vi "Autotest_Instr.vi"(8 "error in (no error)":errorcluster caption="entrée d'erreur (pas d'erreur)", 11 "Class Instrument Multimeter en entrée":refnum<class "Class Instrument Spectrum_Analyser.lvclass">) -> (0 "error out":errorcluster caption="sortie d'erreur", 3 "Class Instrument Multimeter en sortie":refnum<class "Class Instrument Spectrum_Analyser.lvclass">)   [LabVIEW 2020, in "Library Instrument & Equipement.lvlib" / "Library Instruments.lvlib" / "Class Instrument Spectrum_Analyser.lvclass"]
uses:
  Class Instrument Spectrum_Analyser.lvclass
  C:/Users/ngarcin/OneDrive - Altyor/Standard TB/Class/Instrument/Instrument (Default)/Class Instrument (Default).lvclass
  Class Instrument Spectrum_Analyser.lvclass/Class Instrument Spectrum_Analyser.ctl
  Instrument (Default)/Class Instrument (Default).lvclass
  Spectrum Analyser/Class Spectrum Analyser (Default)/Class Spectrum Analyser (Default).lvclass
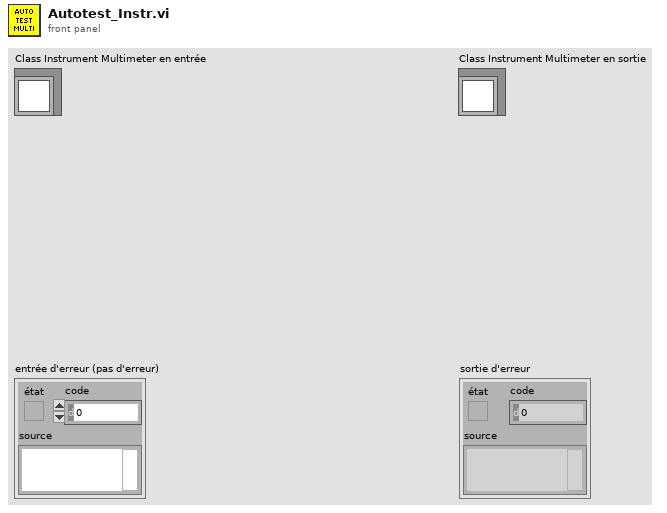
[diagram p1: front panel]
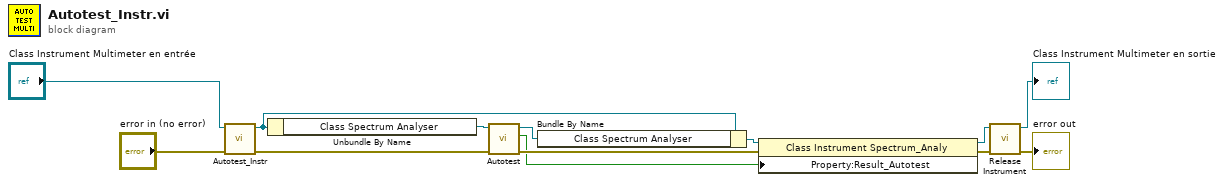
[diagram p0: block diagram]
diagram:
  n1 = call-parent "Autotest_Instr.vi"("error in (no error)"="error in (no error)", "Class Instrument (Default) en entrée"="Class Instrument Multimeter en entrée") -> ("error out"=w5:errorcluster, "Class Instrument (Default) en sortie"=w11:refnum<class "Class Instrument Spectrum_Analyser.lvclass">)  [unwired: 8 in]
  n2 = Unbundle By Name(w11) -> ("Class Spectrum Analyser"=w1:refnum<class "Class Spectrum Analyser (Default).lvclass">)
  n3 = call-dynamic "Autotest.vi"("error in (no error)"=w5, "Class Spectrum Analyser (Default) en entrée"=w1) -> ("error out"=w4:errorcluster, "Autotest Ok ?"=w3:bool, "Class Spectrum Analyser (Default) en sortie"=w2:refnum<class "Class Spectrum Analyser (Default).lvclass">)  [unwired: 7 in]
  n4 = Bundle By Name(cluster=w11, "Class Spectrum Analyser"=w2) -> (w10:refnum<class "Class Instrument Spectrum_Analyser.lvclass">)
  n5 = property class="Class Instrument Spectrum_Analy"(reference=w10, error in=w4, "Property:Result_Autotest"=w3) -> (reference out=w7:refnum<class "Class Instrument Spectrum_Analyser.lvclass">, error out=w9:errorcluster)
  n6 = call-dynamic "Release Instrument.vi"("error in (no error)"=w9, "Class Instrument (Default) en entrée"=w7) -> ("error out"=→"error out":errorcluster, "Class Instrument (Default) en sortie"=→"Class Instrument Multimeter en sortie":refnum<class "Class Instrument Spectrum_Analyser.lvclass">)  [unwired: 8 in]
